vi "Tree Control.vi"() -> ()   [LabVIEW 2020, in "BlueTreeMapExamples OpenSource.lvlib"]
doc: "Demo for the user"
uses:
  BlueTreeMapExamples OpenSource.lvlib
  Typedefs/Tree Node Data.ctl
  Typedefs/Attribute Map.ctl
  Typedefs/Tree Node Data Map.ctl
  Typedefs/Tree Map Export Options.ctl
  Typedefs/Tree Map Export Sorting.ctl
  Typedefs/Sort Type.ctl
  Typedefs/Sort AscDesc.ctl
  Typedefs/AddNodeAction.ctl
  API/New Tree Handle.vi
  API/Add Node.vi
  API/Get Node Data.vi
  API/Get Node Children Data.vi
  API/Get Node Hierarchy Data.vi
  API/Remove Node.vi
  API/Remove Nodes by Filter.vi
  API/Delimited path to array.vi
  API/Tree Map to Tree Control Items.vi
  SubVIs/String to string array.vi
  Classes/Filter Demo/Filter Demo.lvclass
  C:/DSCE code/Open-source/BlueTreeMap/Source/Classes/Filter/Filter.lvclass
  SubVIs/Add Node RecursiveChild.vi
  SubVIs/Get Node Data RecursiveChild.vi
  SubVIs/Get Node Children Data RecursiveChild.vi
  SubVIs/Get Node Hierarchy Data RecursiveChild.vi
  SubVIs/Remove Node RecursiveChild.vi
  SubVIs/Remove Node by Filter RecursiveChild.vi
  SubVIs/Tree Map to Tree Control Items RecursiveChild.vi
  Blue Tree Map OpenSource.lvlib
  C:/DSCE code/Open-source/BlueTreeMap/Source/Examples/Classes/Filter Demo/Filter Demo.lvclass
panel:
  in  "Unit tests":T1(tab)
  out "Node":T2
  out "should be yes 2":bool
  out "children":T4
  out "should be yes 3":bool
  out "Node Hierarchy Data (parent, child)":T2[](array[typedef])
  out "should be yes 4":bool
  out "Node Data before":T2
  out "Node Data after":T2
  out "should be yes 5":bool
  out "should be yes 6":bool
  out "should be yes 7":bool
  out "Node Data 2":T2
  out "should be no 2":bool
  out "should be no 3":bool
  out "before":T2
  out "after":T2
  out "should be no 4":bool
  out "should be yes 8":bool
  out "should be yes 9":bool
  out "should be no 5":bool
  out "Node Data":T2
  out "Node Exists?":bool
  out "Node Path":string="\\Root\\MyNode\\MySubNode"
  in  "Tree Control - Click on the elements":string(tree)="\\Root\\MyNode\\MySubNode"
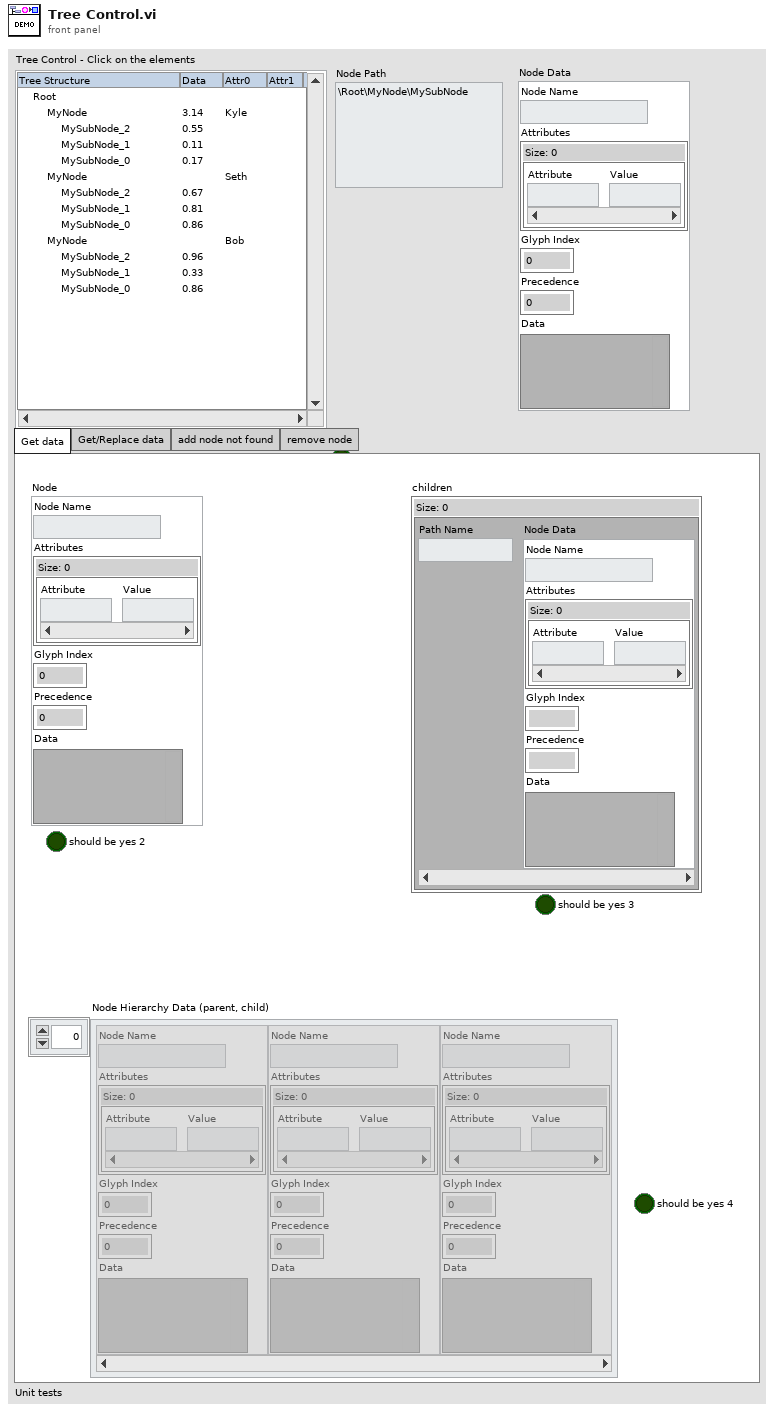
[diagram p1: front panel]
types:
  T1 = enum32{"Get data", "Get/Replace data", "add node not found", "remove node"}
  T2 = typedef "Blue Tree Map OpenSource.lvlib/Tree Node Data.ctl" = cluster{"Node Name":string, "Attributes":T3, "Glyph Index":i32, "Precedence":i32, "Data":variant}
  T3 = typedef "Blue Tree Map OpenSource.lvlib/Attribute Map.ctl" = map{string, string}
  T4 = typedef "Blue Tree Map OpenSource.lvlib/Tree Node Data Map.ctl" = map{string, T2}
  T5 = typedef "Blue Tree Map OpenSource.lvlib/Tree Map Export Options.ctl" = cluster{"Attribute Column Names":string[], "Sort Actions":T6[]}
  T6 = typedef "Blue Tree Map OpenSource.lvlib/Tree Map Export Sorting.ctl" = cluster{"Sort Type":T7, "Order":T8, "Attribute":string}
  T7 = typedef "Blue Tree Map OpenSource.lvlib/Sort Type.ctl" = enum16{"Tree Path Name", "Node Name", "Attribute", "Precedence"}
  T8 = typedef "Blue Tree Map OpenSource.lvlib/Sort AscDesc.ctl" = enum16{"Descending", "Ascending"}
  T9 = typedef "Blue Tree Map OpenSource.lvlib/Tree Map Handle.ctl" = cluster{"Delimiter":string, "Tree Map":T10}
  T10 = typedef "Blue Tree Map OpenSource.lvlib/Tree Map.ctl" = map{string, T11}
  T11 = typedef "Blue Tree Map OpenSource.lvlib/Tree Map Data.ctl" = cluster{"Node Data":T2, "Children":variant}
  T12 = typedef "Blue Tree Map OpenSource.lvlib/AddNodeAction.ctl" = enum16{"Add or Modify Node", "Modify Node only if found"}
  T13 = cluster{"Left Cell String":string, "Child Text":string[], "Child Tag":string, "Item Indent":i32, "Child Only?":bool, "Glyph Index":i32}[]
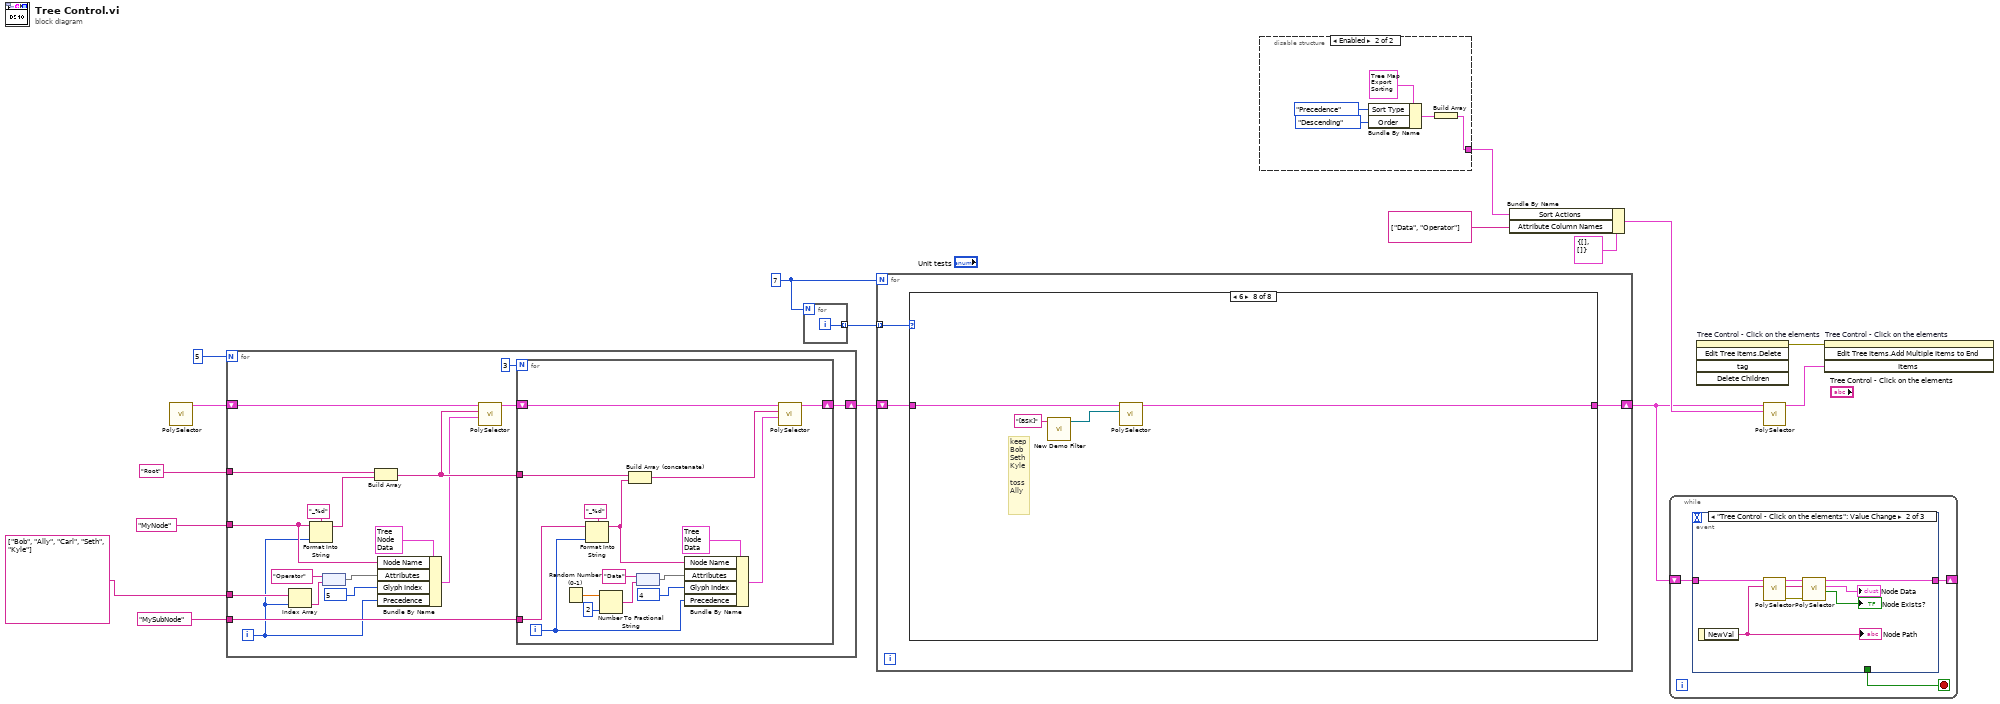
[diagram p0: block diagram]
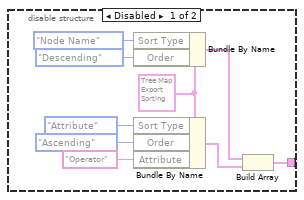
[diagram p2: hidden frame]
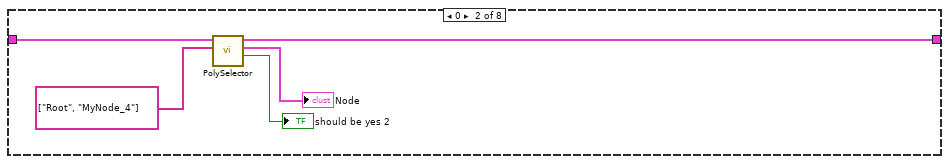
[diagram p4: hidden frame]
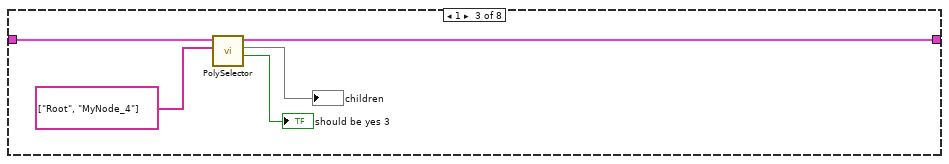
[diagram p5: hidden frame]
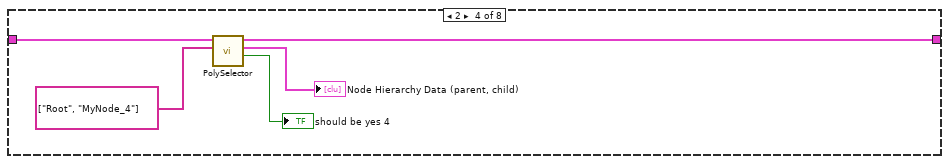
[diagram p6: hidden frame]
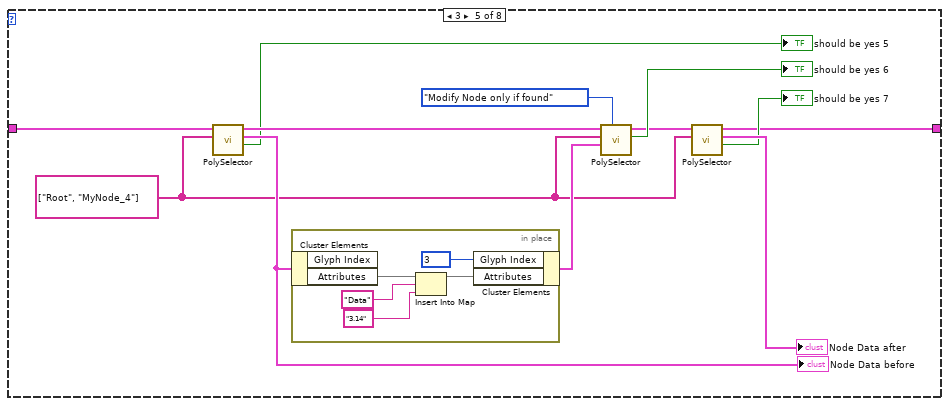
[diagram p7: hidden frame]
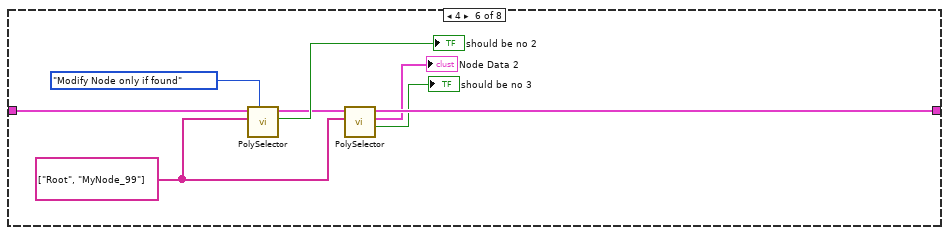
[diagram p8: hidden frame]
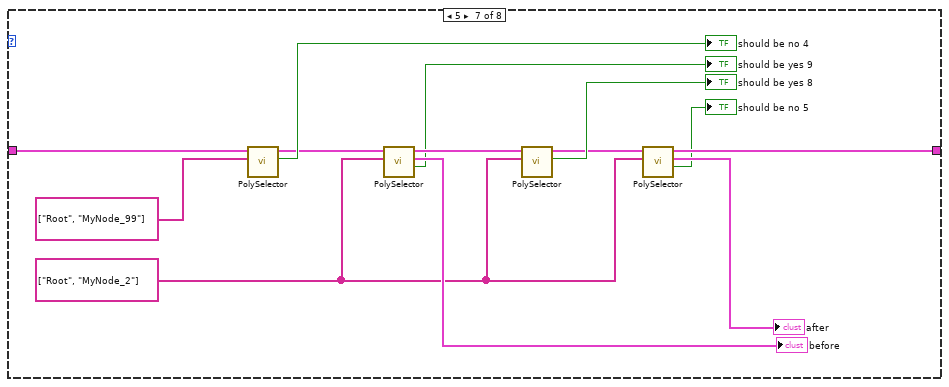
[diagram p9: hidden frame]
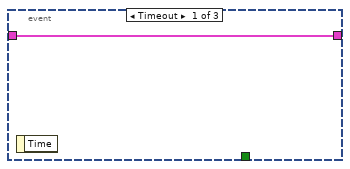
[diagram p10: hidden frame]
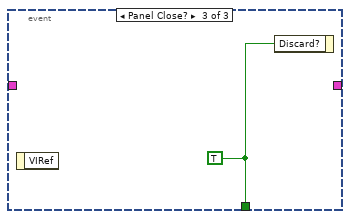
[diagram p11: hidden frame]
diagram:
  w7 = 7
  n1 = call-poly "PolySelector.vi"() -> ("Tree Map Handle Out"=w11:T9)  [unwired: 10 in, 1 out]
  n2 = for {
    N: 5 -> [_]
    tunnel: "MyNode" ("New Node Name") -> [w26]
    shift-right: [w34] -> w9
    shift-left: w11 -> [w23]
    tunnel: "MySubNode" ("New Node Name") -> [w33]
    tunnel: "Root" ("New Root Name") -> [w30]
    tunnel: string[] ["Bob", "Ally", "Carl", "Seth", "Kyle"] -> [w18]
    i -> [w17]
    n3 = Index Array(array=w18, index=w17) -> (element=w19:string)
    n4 = Format Into String(format string="_%d", initial string=w26, w17) -> (resulting string=w28:string)  [unwired: 1 in, 1 out]
    n5 = node("Operator" ("key"), w19) -> (w25:map{string, string})
    n6 = Build Array(w30, w28) -> (w22:string[])
    n7 = Bundle By Name(cluster=T2 {"Node Name"="", "Attributes"={}, "Glyph Index"=0, "Precedence"=0, "Data"=variant} ("Node Data"), "Node Name"=w26, "Attributes"=w25, "Glyph Index"=5, "Precedence"=w17) -> (w21:T2)
    n8 = call-poly "PolySelector.vi"("Node Data"=w21, "New Node Path (parent, child)"=w22, "Tree Map Handle In"=w23) -> ("Tree Map Handle Out"=w20:T9)  [unwired: 6 in, 2 out]
    n9 = for {
      N: 3 -> [_]
      shift-right: [w37] -> w34
      shift-left: w20 -> [w40]
      tunnel: w33 -> [w42]
      tunnel: w22 -> [w48]
      i -> [w35]
      n10 = Random Number (0-1)() -> (number: 0 to 1=w50:dbl)
      n11 = Format Into String(format string="_%d", initial string=w42, w35) -> (resulting string=w36:string)  [unwired: 1 in, 1 out]
      n12 = Number To Fractional String(number=w50, precision (6)=i16 2) -> (F-format string=w43:string)  [unwired: 2 in]
      n13 = Build Array (concatenate)(w48, w36) -> (w39:string[])
      n14 = node("Data" ("key"), w43) -> (w46:map{string, string})
      n15 = Bundle By Name(cluster=T2 {"Node Name"="", "Attributes"={}, "Glyph Index"=0, "Precedence"=0, "Data"=variant} ("Node Data"), "Node Name"=w36, "Attributes"=w46, "Glyph Index"=4, "Precedence"=w35) -> (w38:T2)
      n16 = call-poly "PolySelector.vi"("Node Data"=w38, "New Node Path (parent, child)"=w39, "Tree Map Handle In"=w40) -> ("Tree Map Handle Out"=w37:T9)  [unwired: 6 in, 2 out]
    }
  }
  n17 = for {
    N: w7 -> [_]
    tunnel: [w51] -> w8 mode=indexing
    i -> [w51]
  }
  n18 = for {
    N: w7 -> [_]
    shift-right: [w52] -> w1
    shift-left: w9 -> [w53]
    tunnel: w8 -> [w54] mode=indexing
    n19 = case shown="6" w54 {
      tunnel: w53 -> [w55 w59 w64 w69 w82 w95 w108 w111]
      tunnel: [w55 w58 w63 w68 w71 w90 w99 w109] -> w52
      frame Default {
      }
      frame 0 {
        n20 = call-poly "PolySelector.vi"("Node Path (parent, child)"=string[] ["Root", "MyNode_4"], "Tree Map Handle In"=w59) -> ("Node Exists?"=→"should be yes 2":bool, "Node Data"=→"Node":T2, "Tree Map Handle out"=w58:T9)  [unwired: 6 in, 1 out]
      }
      frame 1 {
        n21 = call-poly "PolySelector.vi"("Node Path (parent, child)"=string[] ["Root", "MyNode_4"], "Tree Map Handle In"=w64) -> ("Node Exists?"=→"should be yes 3":bool, "tree node data map"=→"children":T4, "Tree Map Handle out"=w63:T9)  [unwired: 6 in, 1 out]
      }
      frame 2 {
        n22 = call-poly "PolySelector.vi"("Node Path (parent, child)"=string[] ["Root", "MyNode_4"], "Tree Map Handle In"=w69) -> ("Node Exists?"=→"should be yes 4":bool, "Node Hierarchy Data (parent, child)"=→"Node Hierarchy Data (parent, child)":T2[], "Tree Map Handle out"=w68:T9)  [unwired: 6 in, 1 out]
      }
      frame 3 {
        w74 = string[] ["Root", "MyNode_4"] ("Node Path (parent, child)")
        n23 = call-poly "PolySelector.vi"("Node Path (parent, child)"=w74, "Tree Map Handle In"=w82) -> ("Node Exists?"=→"should be yes 5":bool, "Node Data"=w81:T2, "Tree Map Handle out"=w78:T9)  [unwired: 6 in, 1 out]
        "Node Data before" <- w81
        n24 = in-place {
          n25 = in-place-cluster #1(w81) -> ("Attributes"=w86:T3)  [unwired: 1 out]
          n26 = Insert Into Map(map in=w86, key="Data", value="3.14" ("key")) -> (map out=w85:T3)  [unwired: 2 out]
          n27 = in-place-cluster #1("Glyph Index"=3, "Attributes"=w85) -> (w79:T2)
        }
        n28 = call-poly "PolySelector.vi"("Action (Add)"=AddNodeAction."Modify Node only if found", "Node Data"=w79, "New Node Path (parent, child)"=w74, "Tree Map Handle In"=w78) -> ("Node Data Replaced?"=→"should be yes 6":bool, "Tree Map Handle Out"=w75:T9)  [unwired: 5 in, 1 out]
        n29 = call-poly "PolySelector.vi"("Node Path (parent, child)"=w74, "Tree Map Handle In"=w75) -> ("Node Exists?"=→"should be yes 7":bool, "Node Data"=→"Node Data after":T2, "Tree Map Handle out"=w71:T9)  [unwired: 6 in, 1 out]
      }
      frame 4 {
        w91 = string[] ["Root", "MyNode_99"] ("Node Path (parent, child)")
        n30 = call-poly "PolySelector.vi"("Action (Add)"=AddNodeAction."Modify Node only if found", "New Node Path (parent, child)"=w91, "Tree Map Handle In"=w95) -> ("Node Data Replaced?"=→"should be no 2":bool, "Tree Map Handle Out"=w92:T9)  [unwired: 6 in, 1 out]
        n31 = call-poly "PolySelector.vi"("Node Path (parent, child)"=w91, "Tree Map Handle In"=w92) -> ("Node Exists?"=→"should be no 3":bool, "Node Data"=→"Node Data 2":T2, "Tree Map Handle out"=w90:T9)  [unwired: 6 in, 1 out]
      }
      frame 5 {
        w100 = string[] ["Root", "MyNode_2"] ("Node Path (parent, child)")
        n32 = call-poly "PolySelector.vi"("Node Path (parent, child)"=string[] ["Root", "MyNode_99"], "Tree Map Handle In"=w108) -> ("Node Removed?"=→"should be no 4":bool, "Tree Map Handle Out"=w104:T9)  [unwired: 7 in, 1 out]
        n33 = call-poly "PolySelector.vi"("Node Path (parent, child)"=w100, "Tree Map Handle In"=w104) -> ("Node Exists?"=→"should be yes 9":bool, "Node Data"=→"before":T2, "Tree Map Handle out"=w102:T9)  [unwired: 6 in, 1 out]
        n34 = call-poly "PolySelector.vi"("Node Path (parent, child)"=w100, "Tree Map Handle In"=w102) -> ("Node Removed?"=→"should be yes 8":bool, "Tree Map Handle Out"=w101:T9)  [unwired: 7 in, 1 out]
        n35 = call-poly "PolySelector.vi"("Node Path (parent, child)"=w100, "Tree Map Handle In"=w101) -> ("Node Exists?"=→"should be no 5":bool, "Node Data"=→"after":T2, "Tree Map Handle out"=w99:T9)  [unwired: 6 in, 1 out]
      }
      frame 6 {
        # "keep\nBob\nSeth\nKyle\n\ntoss\nAlly"
        n36 = call "New Demo Filter.vi"("regular expression"="[BSK]") -> ("Filter Demo out"=w110:refnum<class "Filter Demo.lvclass">)  [unwired: 9 in, 1 out]
        n37 = call-poly "PolySelector.vi"("Filter class instructions"=w110, "Tree Map Handle In"=w111) -> ("Tree Map Handle Out"=w109:T9)  [unwired: 8 in, 1 out]
      }
    }
  }
  n38 = disable-structure shown="Enabled" {
    disable-tunnel: [w117 w122] -> w3
    frame Disabled {
      w114 = T6 {"Sort Type"=enum."Tree Path Name", "Order"=enum."Descending", "Attribute"=""} ("Cluster")
      n39 = Bundle By Name(cluster=w114, "Sort Type"=Sort_Type."Node Name" ("Enum"), "Order"=Sort_AscDesc."Descending" ("Enum")) -> (w113:T6)
      n40 = Bundle By Name(cluster=w114, "Sort Type"=Sort_Type."Attribute" ("Enum"), "Order"=Sort_AscDesc."Ascending" ("Enum"), "Attribute"="Operator") -> (w118:T6)
      n41 = Build Array(w113, w118) -> (w117:T6[])
    }
    frame Enabled {
      n42 = Bundle By Name(cluster=T6 {"Sort Type"=enum."Tree Path Name", "Order"=enum."Descending", "Attribute"=""} ("Cluster"), "Sort Type"=Sort_Type."Precedence" ("Enum"), "Order"=Sort_AscDesc."Descending" ("Enum")) -> (w123:T6)
      n43 = Build Array(w123) -> (w122:T6[])
    }
  }
  n44 = Bundle By Name(cluster=T5 {"Attribute Column Names"=[], "Sort Actions"=[]} ("Export Options"), "Sort Actions"=w3, "Attribute Column Names"=string[] ["Data", "Operator"]) -> (w4:T5)
  n45 = while {
    shift-right: [w129] -> _
    shift-left: w1 -> [w128]
    stop <- w127 stop-if-true
    n46 = event shown="[1] \"Tree Control - Click on the elements\": Value Change" {
      selector: _ -> [_ _ _]
      dyn-events: _ -> [_ _ _]
      timeout: _ -> [_ _ _]
      tunnel: [w130 w138 _] -> w129
      tunnel: w128 -> [w130 w135 _]
      tunnel: [_ _ w139] -> w127
      event Timeout {
        n47 = event-data() -> ()  [unwired: 1 in, 1 out]
      }
      event "Tree Control - Click on the elements": Value Change {
        n48 = event-data() -> ("NewVal"=w132:string)  [unwired: 1 in]
        "Node Path" <- w132
        n49 = call-poly "PolySelector.vi"("Node Path Delimited (parent, child)"=w132, "Tree Map Handle In"=w135) -> ("error out"=w131:errorcluster, "Node Path (parent, child)"=w133:string[], "Tree Map Handle out"=w134:T9)  [unwired: 7 in]
        n50 = call-poly "PolySelector.vi"("error in (no error)"=w131, "Node Path (parent, child)"=w133, "Tree Map Handle In"=w134) -> ("Node Exists?"=→"Node Exists?":bool, "Node Data"=→"Node Data":T2, "Tree Map Handle out"=w138:T9)  [unwired: 5 in, 1 out]
      }
      event Panel Close? {
        w139 = TRUE ("Discard?")
        n51 = event-data() -> ()  [unwired: 1 in, 1 out]
        n52 = event-data("Discard?"=w139) -> ()  [unwired: 1 in, 1 out]
      }
    }
  }
  n53 = invoke on="Tree Control - Click on the elements" class="Tree (strict)" method="Edit Tree Items.Delete"() -> (error out=w16:errorcluster)  [unwired: 5 in, 4 out]
  n54 = call-poly "PolySelector.vi"("Export Options"=w4, "Tree Map Handle In"=w1) -> ("Tree Control Items"=w10:T13)  [unwired: 8 in, 1 out]
  n55 = invoke on="Tree Control - Click on the elements" class="Tree (strict)" method="Edit Tree Items.Add Multiple Items to End"(error in=w16, "Items"=w10) -> ()  [unwired: 2 in, 4 out]
